vi "Strategy 2 _ in the making.vi"() -> ()   [LabVIEW 2018]
doc: "This VI is an example of using the PID VI for a PWM application. For a real application all that is needed is the PID VI and the Output to PWM Logic. Together these can be put in the while loop of a real application.\n\nThis example has defaults tuned to the plant."
uses:
  <vilib>/DAQmx/write.llb/DAQmx Write (Digital 1D Bool 1Chan 1Samp).vi
  <vilib>/DAQmx/create/channels.llb/DAQmx Create Channel (DO-Digital Output).vi
  <vilib>/DAQmx/miscellaneous.llb/DAQmx Fill In Error Info.vi
  <vilib>/addons/control/pid/pid.llb/PID (DBL).vi
  <vilib>/addons/control/pid/NI_PID_pid.lvlib
  <vilib>/ptbypt/NI_PtbyPt.lvlib
panel:
  in  "sample length":i32=100
  in  "Slide":dbl(slide) scale=0.0..30.0
  out "Waveform Chart 2":dbl(graph)
  in  "PID gains":T1={"proportional gain (Kc)"=0.1625, "integral time (Ti, min)"=1.25, "derivative time (Td, min)"=0.0} {"derivative time (Td, min)" format="%.3f"; "integral time (Ti, min)" format="%.3f"; "proportional gain (Kc)" format="%.3f"}
  out "PWM Output":bool
  out "Waveform Chart":dbl[][](graph)
  in  "stop":bool
  # "100000 points in buffer"
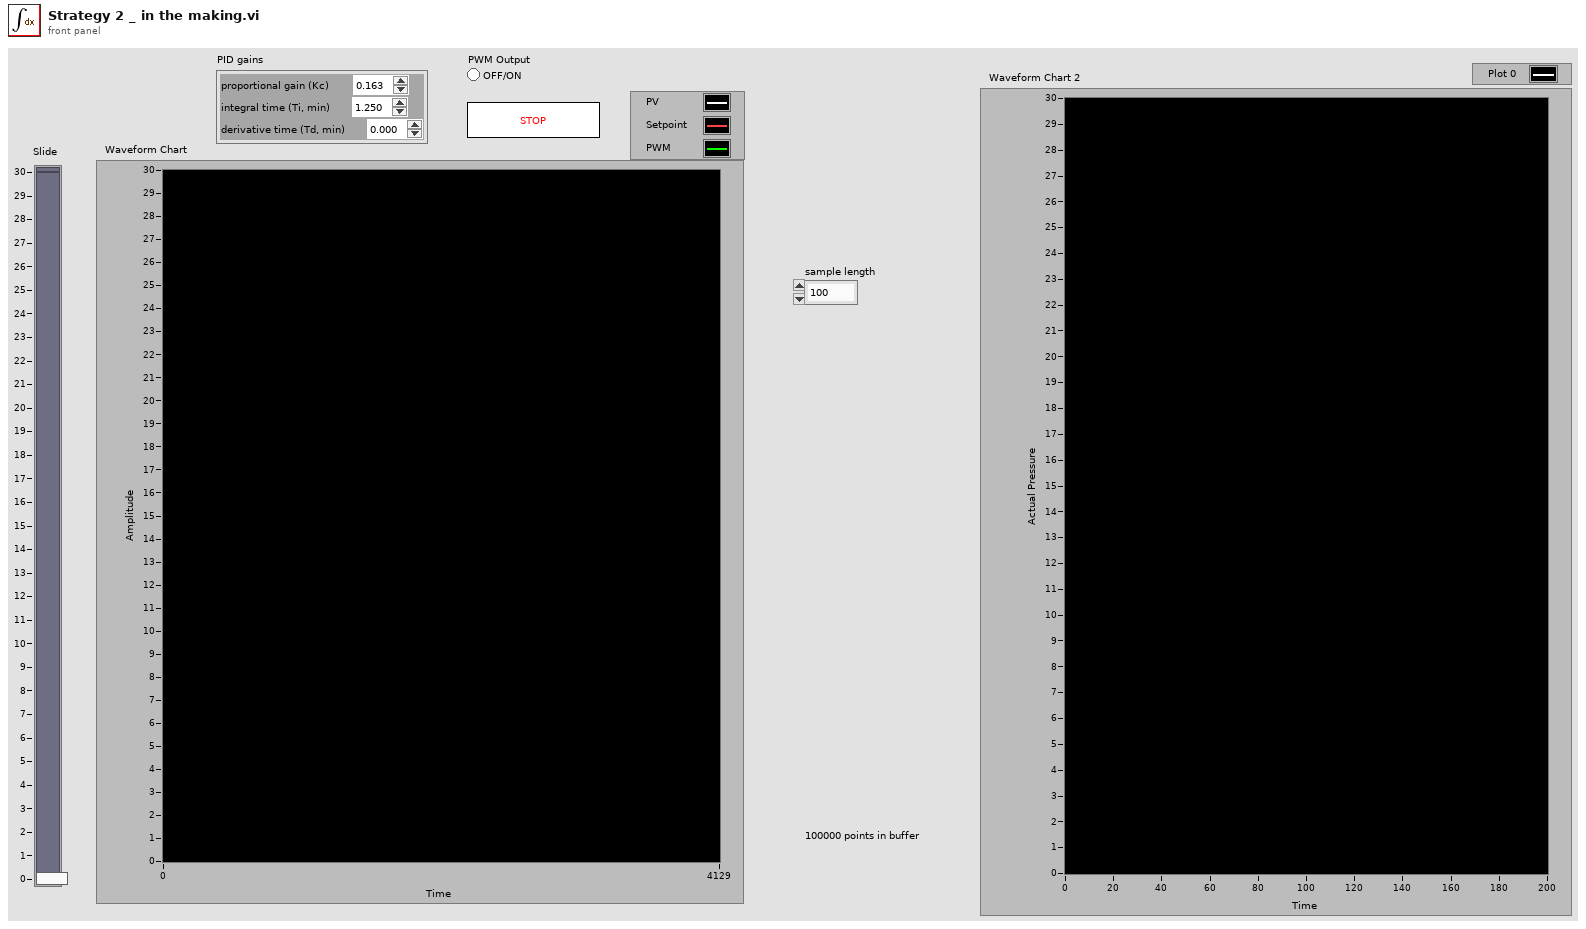
[diagram p1: front panel]
types:
  T1 = cluster{"proportional gain (Kc)":dbl, "integral time (Ti, min)":dbl, "derivative time (Td, min)":dbl}
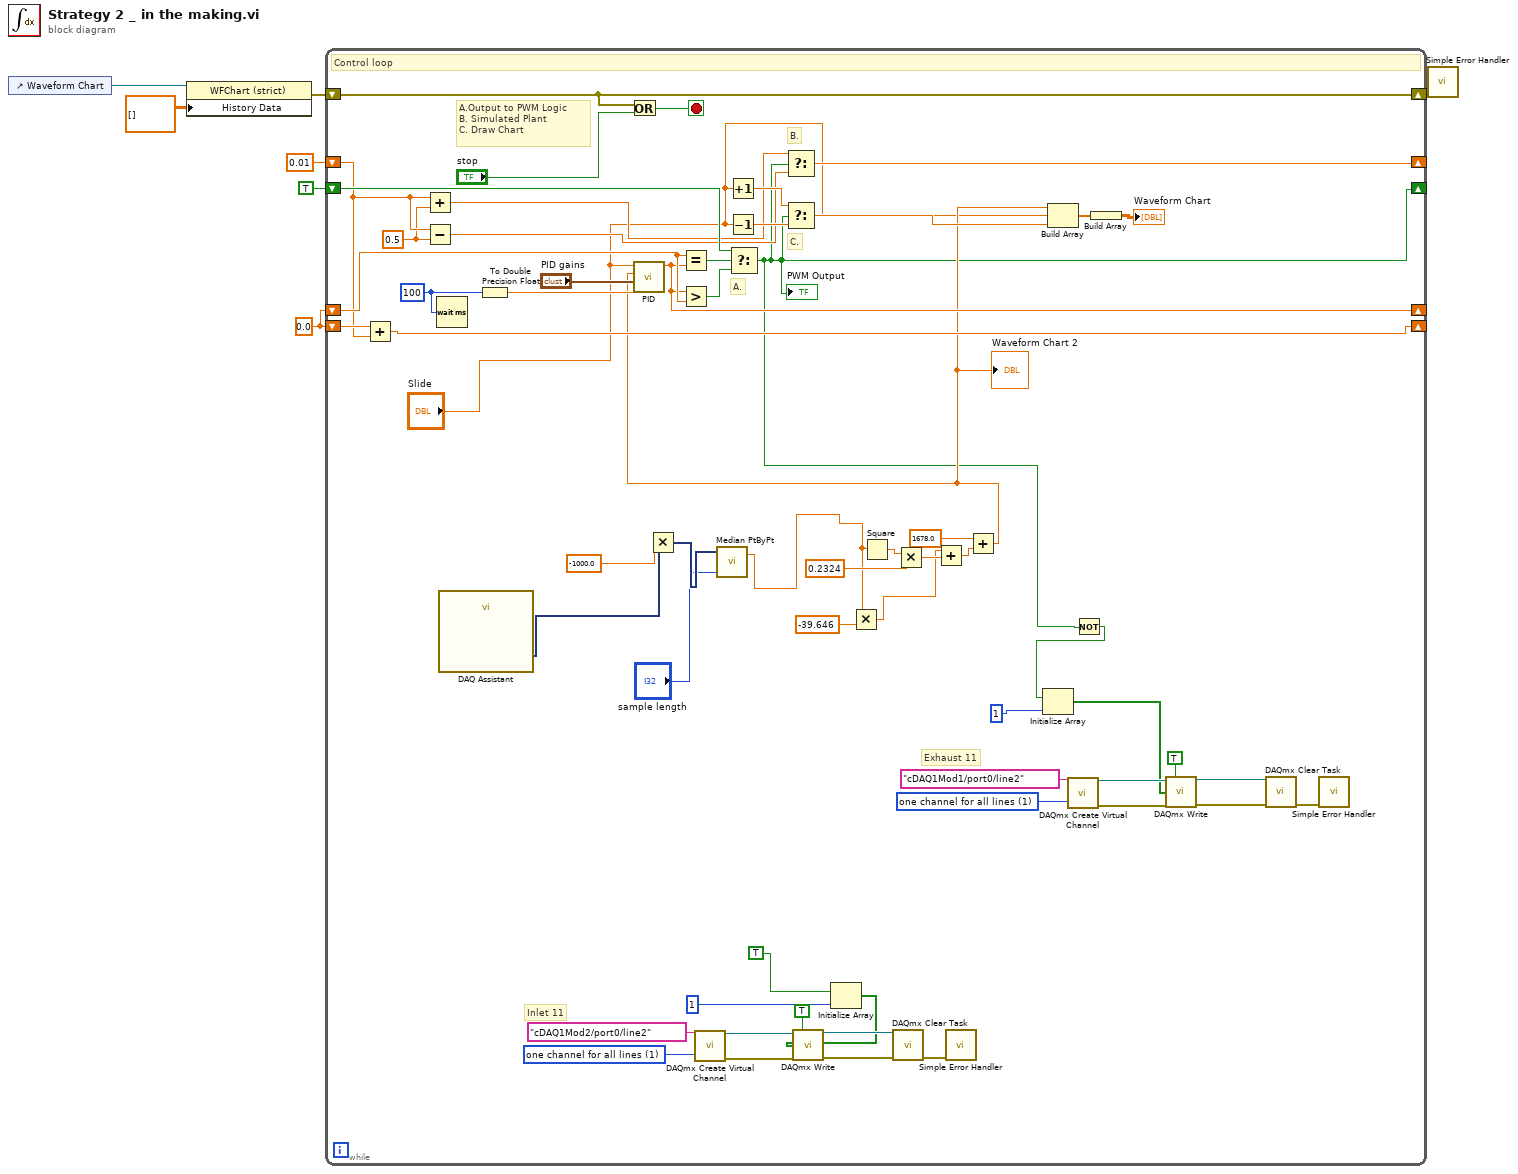
[diagram p0: block diagram]
diagram:
  w6 = 0.0 ("output")
  n1 = control-ref of="Waveform Chart"() -> (w4:refnum<vi>)
  n2 = property class="WFChart (strict)"(reference=w4, "History Data"=dbl[][] []) -> (error out=w3:errorcluster)  [unwired: 1 in, 1 out]
  n3 = while {
    shift-right: [w63] -> _
    shift-left: w6 -> [w64]
    shift-right: [w13] -> _
    shift-left: TRUE -> [w62]
    shift-right: [w60] -> _
    shift-left: w6 -> [w61]
    shift-right: [w58] -> _
    shift-left: 0.01 -> [w59]
    shift-right: [w55] -> w2
    shift-left: w3 -> [w55]
    stop <- w56 stop-if-true
    w18 = 1 items=["one channel for each line", "one channel for all lines"] ("line grouping")
    w36 = 1 items=["one channel for each line", "one channel for all lines"] ("line grouping")
    w47 = 0.5 ("x")
    w65 = u32 100 ("milliseconds to wait")
    # "Exhaust 11"
    # "Inlet 11"
    # "B."
    # "C."
    # "A."
    # "A.Output to PWM Logic \nB. Simulated Plant\nC. Draw Chart"
    # "Control loop"
    n4 = Add(x=w61, y=w59) -> (x+y=w60:dbl)
    n5 = Add(x=w59, y=w47) -> (x+y=w48:dbl)
    n6 = Subtract(x=w59, y=w47) -> (x-y=w46:dbl)
    n7 = Wait (ms)(milliseconds to wait=w65) -> ()  [unwired: 1 out]
    n8 = call "DAQ Assistant"() -> ("data"=w44:dynamicdata)  [unwired: 17 in, 2 out]
    n9 = To Double Precision Float(number=w65) -> (double precision float=w45:dbl)
    n10 = Or(x=w55, y="stop") -> (x .or. y?=w56:bool)
    n11 = Multiply(x=w44, y=-1000.0) -> (x*y=w11:dynamicdata)
    n12 = call-poly <vilib>:"DAQmx Create Virtual Channel.vi"("lines"=tag "cDAQ1Mod2/port0/line2", "line grouping"=w36) -> ("task out"=w38:refnum<k21>, "error out"=w37:errorcluster)  [unwired: 12 in]
    n13 = call <vilib>:"Median PtByPt.vi"("sample length"="sample length", "x"=w11) -> ("median"=w10:dbl)  [unwired: 2 in, 1 out]
    n14 = Increment(x="Slide") -> (x+1=w52:dbl)
    n15 = Decrement(x="Slide") -> (x-1=w51:dbl)
    n16 = Initialize Array(TRUE, 1 ("dimension size")) -> (w33:bool[])
    n17 = call-poly <vilib>:"DAQmx Write.vi"("task/channels in"=w38, "auto start"=TRUE, "data"=w33, "error in"=w37) -> ("task out"=w40:refnum<k21>, "error out"=w41:errorcluster)  [unwired: 9 in, 1 out]
    n18 = Multiply(x=w10, y=-39.646) -> (x*y=w28:dbl)
    n19 = Square(x=w10) -> (x^2=w32:dbl)
    n20 = call <vilib>:"DAQmx Clear Task.vi"("task in"=w40, "error in"=w41) -> ("error out"=w35:errorcluster)  [unwired: 13 in]
    n21 = Multiply(x=w32, y=0.2324) -> (x*y=w29:dbl)
    n22 = Add(x=w28, y=w29) -> (x+y=w27:dbl)
    n23 = call <vilib>:"Simple Error Handler.vi"("error in (no error)"=w35) -> ()  [unwired: 4 in, 5 out]
    n24 = Add(x=1678.0, y=w27) -> (x+y=w25:dbl)
    "Waveform Chart 2" <- w25
    n25 = call-poly <vilib>:"PID.vi"("dt (s)"=w45, "PID gains"="PID gains", "process variable"=w25, "setpoint"="Slide") -> ("output"=w63:dbl)  [unwired: 6 in, 1 out]
    n26 = Equal?(x=w64, y=w63) -> (x = y?=w54:bool)
    n27 = Greater?(x=w63, y=w64) -> (0:w53:bool)
    n28 = Select(t=w62, s=w54, f=w53) -> (s? t:f=w13:bool)
    "PWM Output" <- w13
    n29 = Select(t=w48, s=w13, f=w46) -> (s? t:f=w58:dbl)
    n30 = Select(t=w52, s=w13, f=w51) -> (s? t:f=w50:dbl)
    n31 = Build Array(w25, "Slide", w50) -> (w49:dbl[])
    n32 = call-poly <vilib>:"DAQmx Create Virtual Channel.vi"("lines"=tag "cDAQ1Mod1/port0/line2", "line grouping"=w18) -> ("task out"=w20:refnum<k21>, "error out"=w19:errorcluster)  [unwired: 12 in]
    n33 = Not(x=w13) -> (.not. x?=w12:bool)
    n34 = Initialize Array(w12, 1 ("dimension size")) -> (w15:bool[])
    n35 = Build Array(w49) -> (→"Waveform Chart":dbl[][])
    n36 = call-poly <vilib>:"DAQmx Write.vi"("task/channels in"=w20, "auto start"=TRUE, "data"=w15, "error in"=w19) -> ("task out"=w22:refnum<k21>, "error out"=w23:errorcluster)  [unwired: 9 in, 1 out]
    n37 = call <vilib>:"DAQmx Clear Task.vi"("task in"=w22, "error in"=w23) -> ("error out"=w17:errorcluster)  [unwired: 13 in]
    n38 = call <vilib>:"Simple Error Handler.vi"("error in (no error)"=w17) -> ()  [unwired: 4 in, 5 out]
  }
  n39 = call <vilib>:"Simple Error Handler.vi"("error in (no error)"=w2) -> ()  [unwired: 4 in, 5 out]
